vi "G2CPU Extract Line Profile.vi"(4 "Auto Release Image In (Enabled)":bool=TRUE, 6 "Auto Release Line Indexers":T1={"Auto Release Line Indexers (Enabled)"=TRUE, "Auto Release Keys (Enabled)"=TRUE}, 7 "Out of Range Value":sgl=nan, 8 "error in (no error)":errorcluster, 10 "Line Indexers":T3, 11 "Greyscale Image In":refnum<class "2D Array f32.lvclass">) -> (0 "error out":errorcluster, 3 "Line Profiles Out":T2)   [LabVIEW 2024, in "G2CPU Line Profile.lvlib"]
doc: "Index the input image in order to get the line profiles based on the line indexes provided.\nShould an element out of range it will be substituted by the defined Out of Range Value."
uses:
  G2CPU Line Profile.lvlib
  <vilib>/Natan Biesmans/G2CPU GPU and CPU HPC Toolkit/G2CPU Libraries/Arrays/2DArray/f32/2D Array f32.lvclass
  C:/Program Files/National Instruments/LabVIEW 2025/vi.lib/Natan Biesmans/G2CPU GPU and CPU HPC Toolkit/G2CPU Libraries/Arrays/2DArray/2D Array Prototype.lvclass
  C:/Program Files/National Instruments/LabVIEW 2025/vi.lib/Natan Biesmans/G2CPU GPU and CPU HPC Toolkit/G2CPU Libraries/Arrays/Array/Array Prototype.lvclass
  C:/Program Files/National Instruments/LabVIEW 2025/vi.lib/Natan Biesmans/G2CPU GPU and CPU HPC Toolkit/G2CPU Libraries/Arrays/2DArray/f32/2D Array f32.lvclass
  C:/Program Files/National Instruments/LabVIEW 2025/vi.lib/Natan Biesmans/G2CPU GPU and CPU HPC Toolkit/G2CPU Libraries/Arrays/DataTypes/f32/f32.lvclass
  <vilib>/Natan Biesmans/G2CPU GPU and CPU HPC Toolkit/G2CPU Libraries/Arrays/1DArray/f32/1D Array f32.lvclass
  C:/Program Files/National Instruments/LabVIEW 2025/vi.lib/Natan Biesmans/G2CPU GPU and CPU HPC Toolkit/G2CPU Libraries/Arrays/1DArray/1D Array Prototype.lvclass
  C:/Program Files/National Instruments/LabVIEW 2025/vi.lib/Natan Biesmans/G2CPU GPU and CPU HPC Toolkit/G2CPU Libraries/Arrays/1DArray/f32/1D Array f32.lvclass
  8151d9b9-df04-4fa2-a4dc-4c7bad1d0c96.vi
  6a31e8c2-bae3-46ba-b70a-58cc8e0c847c.vi
  e10e66f0-73c2-4ec3-8fb8-7ad0e5b8f3d0.vi
  <vilib>/Natan Biesmans/G2CPU GPU and CPU HPC Toolkit/G2CPU Libraries/Arrays/Array/Array Prototype.lvclass
  <vilib>/Natan Biesmans/G2CPU GPU and CPU HPC Toolkit/ArrayFire Driver/TypeDefs/Dim4.ctl
  <vilib>/Natan Biesmans/G2CPU GPU and CPU HPC Toolkit/ArrayFire Driver/AF.lvlib
  87b054ba-0c2d-4e34-b65d-2938af21a854.vi
  e5c67453-36f4-4b4b-8c3f-eb38d0038472.vi
  698ed075-5c63-4b85-b6d5-f4acdeaa938e.vi
  4d1ec8f5-56bb-4b65-bfee-e2770057249d.vi
  <vilib>/Natan Biesmans/G2CPU GPU and CPU HPC Toolkit/G2CPU Libraries/Arrays/1DArray/u32/1D Array u32.lvclass
  e389581e-2be3-4b88-b7f2-c15ded704882.vi
  <vilib>/Natan Biesmans/G2CPU GPU and CPU HPC Toolkit/G2CPU Libraries/Arrays/2DArray/u32/2D Array u32.lvclass
  e0a14033-9bac-4334-9c94-5d62948e0446.vi
  1a1d34bd-cc7a-4492-9572-715fec3c383f.vi
  2419fe12-094d-4bc3-8916-e4052a89274d.vi
  414be421-639e-49ae-9722-7b7ed246bfa1.vi
  <vilib>/Natan Biesmans/G2CPU GPU and CPU HPC Toolkit/G2CPU Libraries/Arrays/2DArray/s32/2D Array s32.lvclass
  c31e3477-3027-4a8c-840d-6d380c6ce67e.vi
  7b908a32-4f4a-4d1d-915c-c85414a39aa6.vi
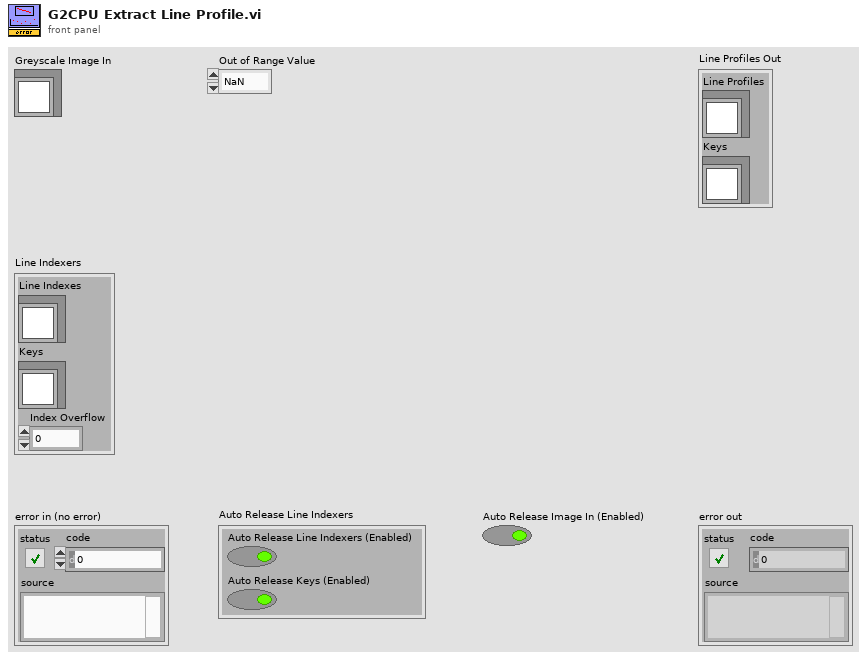
[diagram p1: front panel]
types:
  T1 = cluster{"Auto Release Line Indexers (Enabled)":bool, "Auto Release Keys (Enabled)":bool}
  T2 = cluster{"Line Profiles":refnum<class "2D Array f32.lvclass">, "Keys":refnum<class "2D Array u32.lvclass">}
  T3 = cluster{"Line Indexes":refnum<class "2D Array f32.lvclass">, "Keys":refnum<class "2D Array u32.lvclass">, "Index Overflow":u64}
  T4 = typedef "AF.lvlib/Dim4.ctl" = cluster{"Dim 0":u64, "Dim 1":u64, "Dim 2":u64, "Dim 3":u64}
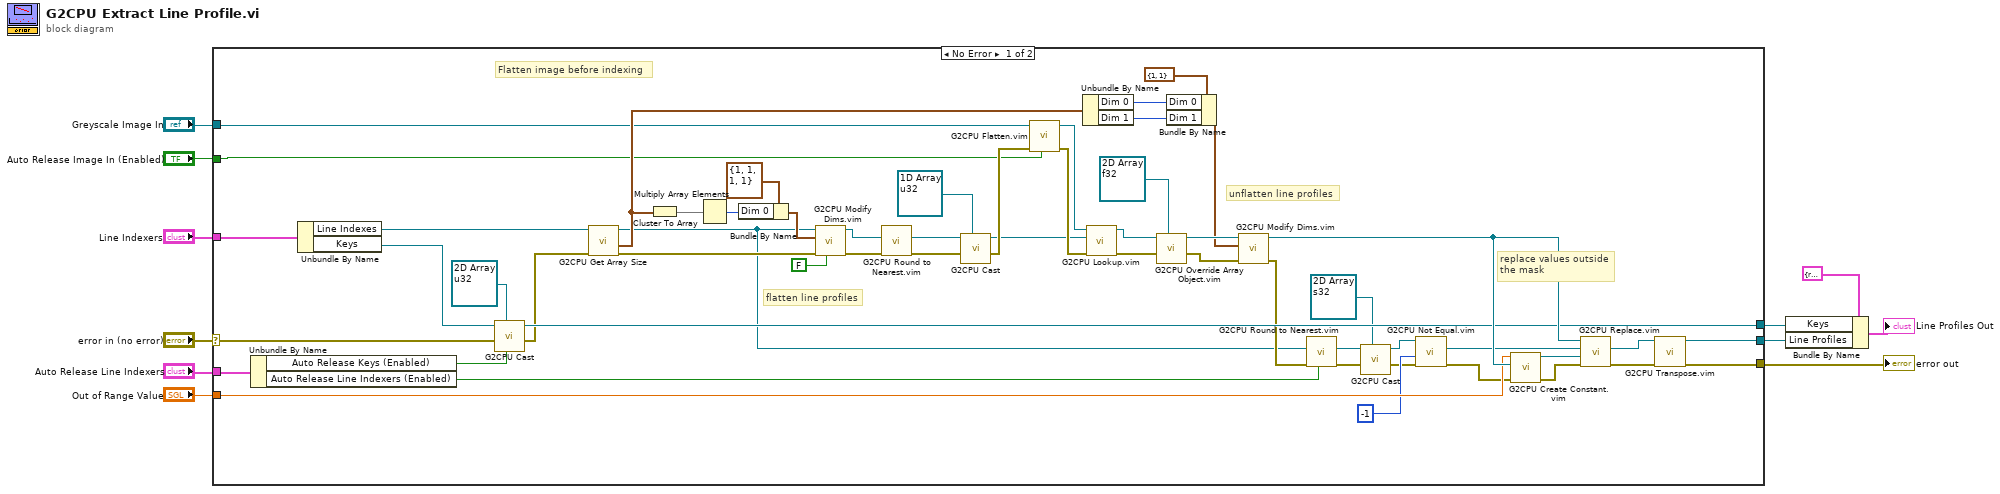
[diagram p0: block diagram]
diagram:
  n1 = case shown="No Error" "error in (no error)" {
    selector: "error in (no error)" -> [w32 w67]
    tunnel: "Greyscale Image In" -> [w27 _]
    tunnel: [w51 _] -> w3
    tunnel: [w50 w67] -> w10
    tunnel: "Auto Release Image In (Enabled)" -> [w26 _]
    tunnel: "Out of Range Value" -> [w63 _]
    tunnel: "Line Indexers" -> [w47 _]
    tunnel: "Auto Release Line Indexers" -> [w45 _]
    tunnel: [w33 _] -> w2
    frame No Error {
      # "replace values outside\nthe mask"
      # "Flatten image before indexing"
      # "flatten line profiles"
      # "unflatten line profiles"
      n2 = Unbundle By Name(w45) -> ("Auto Release Keys (Enabled)"=w29:bool, "Auto Release Line Indexers (Enabled)"=w12:bool)
      n3 = Unbundle By Name(w47) -> ("Line Indexes"=w36:refnum<class "2D Array f32.lvclass">, "Keys"=w34:refnum<class "2D Array u32.lvclass">)
      n4 = call "G2CPU Cast"("Auto Release Low (Enabled)"=w29, "Datatype Prototype"=refnum<class "2D Array u32.lvclass"> refnum ("Keys"), "error in (no error)"=w32, "Array In"=w34) -> ("error out"=w31:errorcluster, "Array Out"=w33:refnum<class "2D Array u32.lvclass">)  [unwired: 6 in]
      n5 = call <vilib>:"G2CPU Get Array Size.vi"("error in (no error)"=w31, "Array in"=w36) -> ("error out"=w55:errorcluster, "Array Size"=w39:T4, "Array out"=w15:refnum<class "2D Array f32.lvclass">)  [unwired: 6 in, 1 out]
      n6 = Cluster To Array(cluster=w39) -> (array=w58:u64[])
      n7 = Multiply Array Elements(1:w58) -> (0:w57:u64)
      n8 = Bundle By Name(cluster=T4 {"Dim 0"=1, "Dim 1"=1, "Dim 2"=1, "Dim 3"=1} ("dims"), "Dim 0"=w57) -> (w56:T4)
      n9 = call "G2CPU Modify Dims.vim"("Auto Release (Enabled)"=FALSE, "error in (no error)"=w55, "dims"=w56, "Array In"=w15) -> ("error out"=w24:errorcluster, "Array out"=w25:refnum<class "4D Array f32.lvclass">)  [unwired: 6 in]
      n10 = call "G2CPU Round to Nearest.vim"("error in (no error)"=w24, "Array in"=w25) -> ("error out"=w23:errorcluster, "Array Result"=w20:refnum<class "4D Array f32.lvclass">)  [unwired: 8 in]
      n11 = call "G2CPU Cast"("Datatype Prototype"=refnum<class "1D Array u32.lvclass"> refnum ("Array out"), "error in (no error)"=w23, "Array In"=w20) -> ("error out"=w28:errorcluster, "Array Out"=w22:refnum<class "1D Array u32.lvclass">)  [unwired: 7 in]
      n12 = call "G2CPU Flatten.vim"("Auto Release (Enabled)"=w26, "error in (no error)"=w28, "Array In"=w27) -> ("error out"=w30:errorcluster, "Array out"=w44:refnum<class "1D Array f32.lvclass">)  [unwired: 7 in]
      n13 = Unbundle By Name(w39) -> ("Dim 0"=w38:u64, "Dim 1"=w37:u64)
      n14 = call "G2CPU Lookup.vim"("error in (no error)"=w30, "Indices (1D)"=w22, "Array In"=w44) -> ("error out"=w43:errorcluster, "Indexed Array"=w42:refnum<class "1D Array f32.lvclass">)  [unwired: 7 in]
      n15 = call "G2CPU Override Array Object.vim"("New Array Type"=refnum<class "2D Array f32.lvclass"> refnum ("Array Out"), "error in (no error)"=w43, "To Override Array"=w42) -> ("error out"=w54:errorcluster, "Overriden Array (inplace)"=w62:refnum<class "2D Array f32.lvclass">)  [unwired: 7 in]
      n16 = Bundle By Name(cluster=cluster{"Dim 0":u64, "Dim 1":u64} {"Dim 0"=1, "Dim 1"=1} ("Array Size"), "Dim 0"=w38, "Dim 1"=w37) -> (w40:cluster{"Dim 0":u64, "Dim 1":u64})
      n17 = call "G2CPU Modify Dims.vim"("error in (no error)"=w54, "dims"=w40, "Array In"=w62) -> ("error out"=w16:errorcluster, "Array out"=w66:refnum<class "2D Array f32.lvclass">)  [unwired: 7 in]
      n18 = call "G2CPU Round to Nearest.vim"("Auto Release (Enabled)"=w12, "error in (no error)"=w16, "Array in"=w15) -> ("error out"=w17:errorcluster, "Array Result"=w13:refnum<class "2D Array f32.lvclass">)  [unwired: 7 in]
      n19 = call "G2CPU Cast"("Datatype Prototype"=refnum<class "2D Array s32.lvclass"> refnum ("Array out"), "error in (no error)"=w17, "Array In"=w13) -> ("error out"=w19:errorcluster, "Array Out"=w18:refnum<class "2D Array s32.lvclass">)  [unwired: 7 in]
      n20 = call "G2CPU Not Equal.vim"("error in (no error)"=w19, "Array rhs"=-1, "Array lhs"=w18) -> ("error out"=w49:errorcluster, "Array Result"=w48:refnum<class "2D Array binary.lvclass">)  [unwired: 7 in]
      n21 = call "G2CPU Create Constant.vim"("error in (no error)"=w49, "Size"=w66, "val"=w63) -> ("error out"=w64:errorcluster, "object out"=w65:refnum<class "2D Array f32.lvclass">)  [unwired: 7 in]
      n22 = call "G2CPU Replace.vim"("error in (no error)"=w64, "To Replace Values Array or scalar Value"=w65, "Replace  Condition"=w48, "Array In"=w66) -> ("error out"=w52:errorcluster, "Array out (same as in)"=w53:refnum<class "2D Array f32.lvclass">)  [unwired: 6 in]
      n23 = call "G2CPU Transpose.vim"("error in (no error)"=w52, "Array In"=w53) -> ("error out"=w50:errorcluster, "Array out"=w51:refnum<class "2D Array f32.lvclass">)  [unwired: 8 in]
    }
    frame Error {
    }
  }
  "error out" <- w10
  n24 = Bundle By Name(cluster=T2 {"Line Profiles"=refnum, "Keys"=refnum} ("Line Profiles Out"), "Keys"=w2, "Line Profiles"=w3) -> (→"Line Profiles Out":T2)
